vi "Error-Query.vi"(8 "error in (no error)":errorcluster {"code" format="%.0x"}, 11 "instrument handle":refnum<k15>) -> (0 "error out":errorcluster {"code" format="%.0x"}, 1 "error message":string, 2 "error code":i32 format="%.0g", 3 "instrument handle out":refnum<k15>)   [LabVIEW 2020, in "Keysight DAQ970.lvlib"]
doc: "Queries the instrument and returns instrument specific error information. This function can be used when QueryInstrumentStatus is True to retrieve error details when the driver detects an instrument error."
uses:
  Keysight DAQ970.lvlib
  KtDAQ970.dll
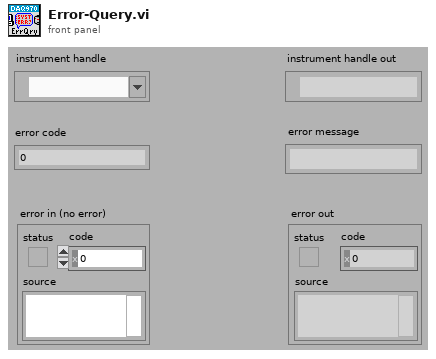
[diagram p1: front panel]
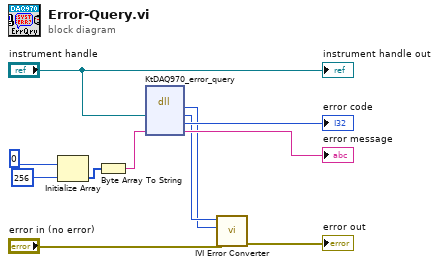
[diagram p0: block diagram]
diagram:
  n1 = Initialize Array(u8 0, 256) -> (w8:u8[])
  n2 = Byte Array To String(unsigned byte array=w8) -> (string=w6:string)
  n3 = dll-call lib="KtDAQ970**.dll" fn="KtDAQ970_error_query" ("LabVIEW:IviDmm_error_query")("instrument handle"="instrument handle", "error message"=w6) -> ("Status"=w1:i32, "instrument handle"=w4:u32, "error code"=→"error code":i32, "error message"=→"error message":string)  [unwired: 3 in, 3 out]
  n4 = call "IVI Error Converter.vi"("error in (no error)"="error in (no error)", "IVI error code (0)"=w1, "instrument handle"=w4) -> ("error out"=→"error out":errorcluster)  [unwired: 7 in, 1 out]
  "instrument handle out" <- "instrument handle"
